vi "PolytecResult.vi"(10 "Bilans[0]":i8, 11 "Bilan_General":i8) -> (1 "Result":string)   [LabVIEW 2020]
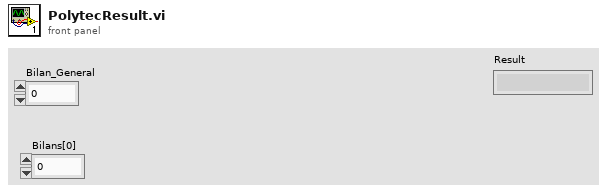
[diagram p1: front panel]
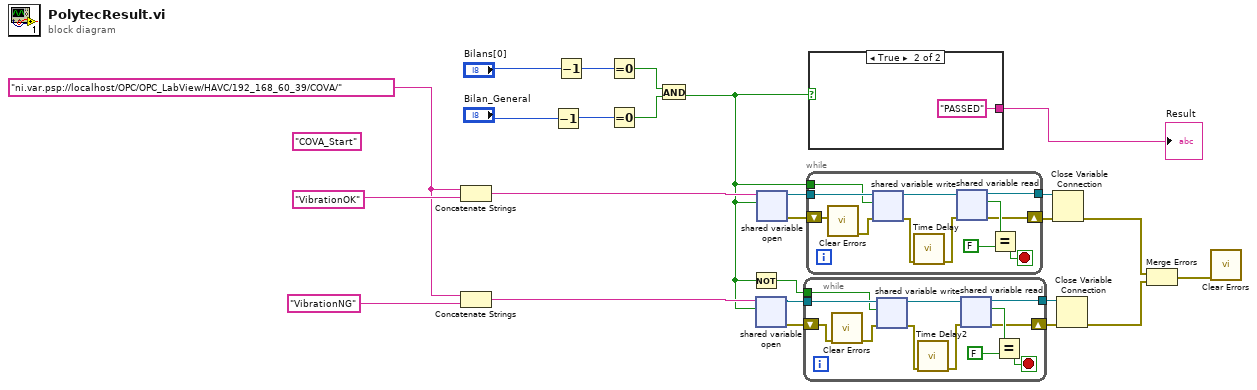
[diagram p0: block diagram]
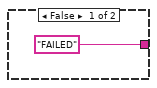
[diagram p2: hidden frame]
diagram:
  (unwired) "COVA_Start"
  w24 = "ni.var.psp://localhost/OPC/OPC_LabView/HAVC/192_168_60_39/COVA/" ("string")
  n1 = Concatenate Strings(w24, "VibrationOK") -> (w15:string)
  n2 = Concatenate Strings(w24, "VibrationNG" ("string")) -> (w14:string)
  n3 = Decrement(x="Bilan_General") -> (x-1=w19:i8)
  n4 = Decrement(x="Bilans[0]") -> (x-1=w20:i8)
  n5 = Equal To 0?(x=w20) -> (x = 0?=w17:bool)
  n6 = Equal To 0?(x=w19) -> (x = 0?=w18:bool)
  n7 = And(x=w17, y=w18) -> (x .and. y?=w1:bool)
  n8 = Not(x=w1) -> (.not. x?=w2:bool)
  n9 = shared-variable-open(w14, w1) -> (w6:refnum<k21>, w5:errorcluster)  [unwired: 2 in]
  n10 = shared-variable-open(w15, w1) -> (w10:refnum<k21>, w3:errorcluster)  [unwired: 2 in]
  n11 = while {
    tunnel: [w32] -> w7
    tunnel: w6 -> [w31]
    tunnel: w2 -> [w27]
    shift-right: [w26] -> w4
    shift-left: w5 -> [w28]
    stop <- w30 stop-if-true
    n12 = call <vilib>:"Clear Errors.vi"("error in (no error)"=w28) -> ("error out"=w33:errorcluster)  [unwired: 5 in, 1 out]
    n13 = shared-variable-write(w31, w33, w27) -> (w35:refnum<k21>, w36:errorcluster)
    n14 = call "Time Delay2"("error in (no error)"=w36) -> ("error out"=w37:errorcluster)  [unwired: 10 in]
    n15 = shared-variable-read(w35, w37) -> (w32:refnum<k21>, w26:errorcluster, w29:bool)  [unwired: 1 out]
    n16 = Equal?(x=w29, y=FALSE) -> (x = y?=w30:bool)
  }
  n17 = while {
    tunnel: w10 -> [w46]
    tunnel: w1 -> [w45]
    tunnel: [w40] -> w8
    shift-right: [w41] -> w9
    shift-left: w3 -> [w38]
    stop <- w44 stop-if-true
    n18 = call <vilib>:"Clear Errors.vi"("error in (no error)"=w38) -> ("error out"=w39:errorcluster)  [unwired: 5 in, 1 out]
    n19 = shared-variable-write(w46, w39, w45) -> (w47:refnum<k21>, w48:errorcluster)
    n20 = call "Time Delay"("error in (no error)"=w48) -> ("error out"=w49:errorcluster)  [unwired: 10 in]
    n21 = shared-variable-read(w47, w49) -> (w40:refnum<k21>, w41:errorcluster, w43:bool)  [unwired: 1 out]
    n22 = Equal?(x=w43, y=FALSE) -> (x = y?=w44:bool)
  }
  n23 = case shown="True" w1 {
    tunnel: ["FAILED" ("Result") "PASSED" ("Result")] -> w16
    frame False {
    }
    frame True {
    }
  }
  "Result" <- w16
  n24 = Close Variable Connection(8:w9, 11:w8) -> (0:w12:errorcluster)
  n25 = Close Variable Connection(8:w4, 11:w7) -> (0:w13:errorcluster)
  n26 = Merge Errors(w12, w13) -> (w11:errorcluster)
  n27 = call <vilib>:"Clear Errors.vi"("error in (no error)"=w11) -> ()  [unwired: 5 in, 2 out]
